vi "Simple TCP - Client.vi"() -> ()   [LabVIEW 2014]
doc: "Demonstrates how to open a connection to an TCP server, read the data being sent, and display the data on a chart. This VI is designed to stop if the TCP connection is terminated."
panel:
  in  "Send":bool
  in  "TCP Send":string
  out "TCP Received":string
  in  "Stop":bool
  # "Overview: Demonstrates the use of the TCP functions to connect to a TCP server VI and receive data.\nInstructions:\n1. Ensure Simple TCP - Server.vi is already running.\n2. Run the VI.\n3. Click Stop to stop the VI. Note that if you stop the server VI, this VI will stop automatically."
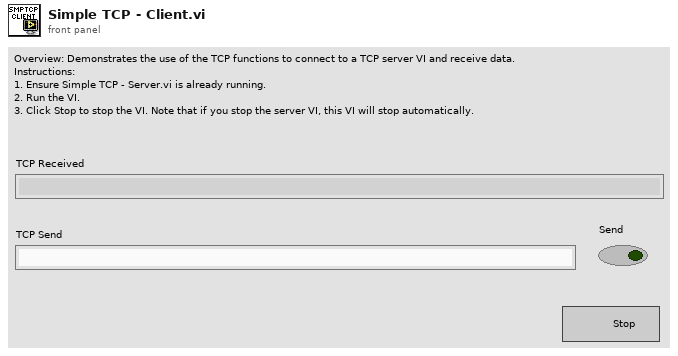
[diagram p1: front panel]
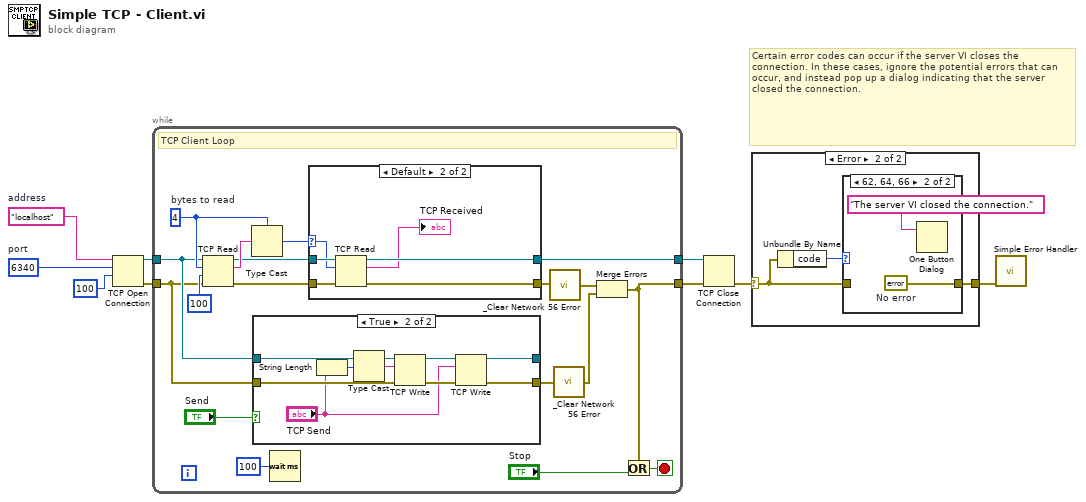
[diagram p0: block diagram]
diagram:
  w4 = u16 6340  # port
  w5 = "localhost"  # address
  # "Certain error codes can occur if the server VI closes the connection. In these cases, ignore the potential errors that can occur, and instead pop up a dialog indicating that the server closed the connection."
  n1 = TCP Open Connection(address=w5, remote port or service name=w4, timeout ms (60000)=100 ("timeout ms (25000)")) -> (connection ID=w9:refnum<k5>, error out=w8:errorcluster)  [unwired: 2 in]
  n2 = while {
    tunnel: w8 -> [w14]
    tunnel: w9 -> [w15]
    tunnel: [w12] -> w2
    tunnel: [w11] -> w3
    stop <- w22 stop-if-true
    w24 = 4  # bytes to read
    # "TCP Client Loop"
    n3 = TCP Read(connection ID=w15, bytes to read=w24, error in (no error)=w14, 9:100 ("timeout ms (25000)")) -> (connection ID out=w26:refnum<k5>, data out=w27:string, error out=w25:errorcluster)  [unwired: 1 in]
    n4 = Type Cast(type=w24, x=w27) -> (*(type *) &x=w20:i32)
    n5 = case shown="True" "Send" {
      tunnel: w15 -> [w29 w38]
      tunnel: w14 -> [w28 w35]
      tunnel: [w28 w34] -> w17
      tunnel: [w29 w33] -> _
      frame False {
      }
      frame True {
        n6 = String Length(string="TCP Send") -> (length=w32:i32)
        n7 = Type Cast(x=w32) -> (*(type *) &x=w30:string)  [unwired: 1 in]
        n8 = TCP Write(connection ID=w38, data in=w30, error in (no error)=w35) -> (connection ID out=w37:refnum<k5>, error out=w36:errorcluster)  [unwired: 1 in, 1 out]
        n9 = TCP Write(connection ID=w37, data in="TCP Send", error in (no error)=w36) -> (connection ID out=w33:refnum<k5>, error out=w34:errorcluster)  [unwired: 1 in, 1 out]
      }
    }
    n10 = Wait (ms)(milliseconds to wait=u32 100) -> ()  [unwired: 1 out]
    n11 = case shown="Default" w20 {
      selector: w20 -> [_ w42]
      tunnel: w26 -> [w40 w46]
      tunnel: w25 -> [w39 w45]
      tunnel: [w40 w44] -> w12
      tunnel: [w39 w43] -> w13
      frame ..0 {
        # "The server has not written any data"
      }
      frame Default {
        n12 = TCP Read(connection ID=w46, bytes to read=w42, error in (no error)=w45) -> (connection ID out=w44:refnum<k5>, data out=→"TCP Received":string, error out=w43:errorcluster)  [unwired: 2 in]
      }
    }
    n13 = call "_Clear Network 56 Error.vi"("error in (no error)"=w13) -> ("error out"=w10:errorcluster)  [unwired: 4 in]
    n14 = call "_Clear Network 56 Error.vi"("error in (no error)"=w17) -> ("error out"=w16:errorcluster)  [unwired: 4 in]
    n15 = Merge Errors(w10, w16) -> (w11:errorcluster)
    n16 = Or(x=w11, y="Stop") -> (x .or. y?=w22:bool)
  }
  n17 = TCP Close Connection(connection ID=w2, error in (no error)=w3) -> (error out=w7:errorcluster)  [unwired: 1 in, 1 out]
  n18 = case shown="Error" w7 {
    selector: w7 -> [w47 w49]
    tunnel: [w47 w48] -> w6
    frame No Error {
    }
    frame Error {
      n19 = Unbundle By Name(w49) -> ("code"=w50:i32)
      n20 = case shown="62, 64, 66" w50 {
        tunnel: w49 -> [w51 _]
        tunnel: [w51 w53] -> w48
        frame Default {
        }
        frame 62, 64, 66 {
          w53 = errorcluster {"status"=FALSE, "code"=0, "source"=""}  # No error
          n21 = One Button Dialog(message="The server VI closed the connection." ("Server Closed")) -> ()  [unwired: 1 in, 1 out]
        }
      }
    }
  }
  n22 = call <vilib>:"Simple Error Handler.vi"("error in (no error)"=w6) -> ()  [unwired: 4 in, 5 out]
